vi "svpo_Average Array (complex).vi"(6 "averages completed in":dbl, 7 "restart averaging":bool, 8 "exponential weight (10 %)":dbl=10.0 min=0.0 max=100.0 step=5.0, 9 "weighting mode":enum16{"Linear", "Exponential"}(ring), 10 "array":cdb[](array[numeric]) format="%.2p", 11 "previous average array":cdb[](array[numeric]) format="%.2p") -> (2 "averages completed out":dbl, 3 "average array":cdb[](array[numeric]) format="%.2p")   [LabVIEW 2017]
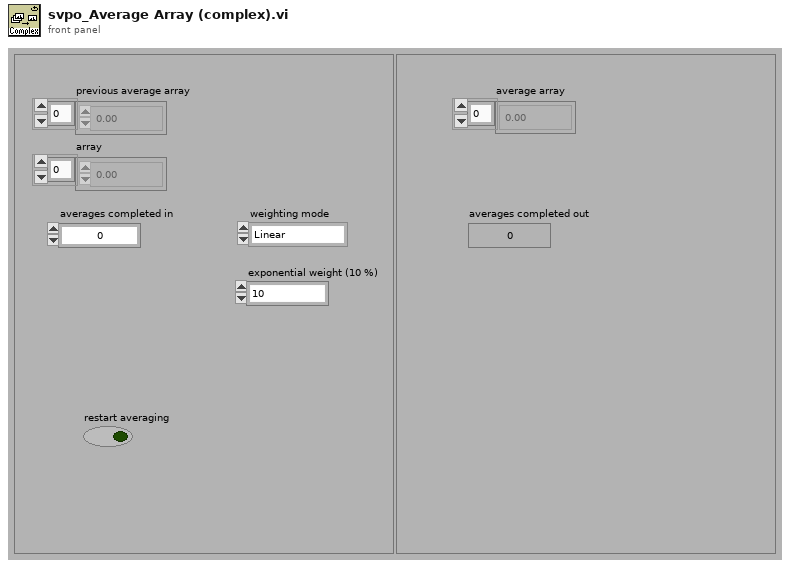
[diagram p1: front panel]
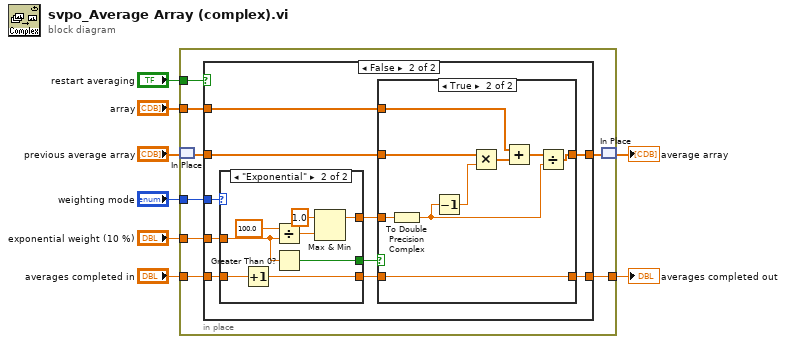
[diagram p0: block diagram]
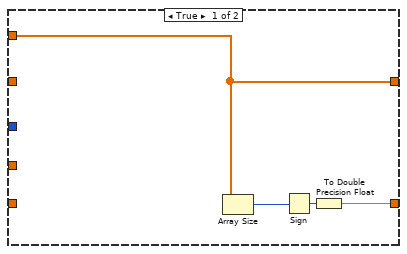
[diagram p2: hidden frame]
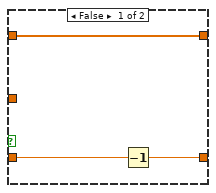
[diagram p3: hidden frame]
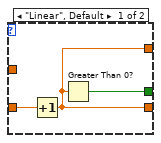
[diagram p4: hidden frame]
diagram:
  n1 = in-place {
    in-place-border: "array" -> [w16]
    in-place-border: "exponential weight (10 %)" -> [w15]
    in-place-border: "weighting mode" -> [w14]
    in-place-border: "averages completed in" -> [w13]
    in-place-border: [w12] -> w4
    in-place-border: "restart averaging" -> [w11]
    n2 = in-place-match #1("previous average array") -> (w10:cdb[])
    n3 = case shown="False" w11 {
      tunnel: w16 -> [w20 w29]
      tunnel: [w20 w24] -> w9
      tunnel: [w19 w22] -> w12
      tunnel: w10 -> [_ w28]
      tunnel: w15 -> [_ w27]
      tunnel: w14 -> [_ w26]
      tunnel: w13 -> [_ w25]
      frame True {
        n4 = Array Size(array=w20) -> (size(s)=w18:i32)
        n5 = Sign(1:w18) -> (0:w17:i32)
        n6 = To Double Precision Float(number=w17) -> (double precision float=w19:dbl)
      }
      frame False {
        n7 = case shown="\"Exponential\"" w26 {
          tunnel: w25 -> [w45 w52]
          tunnel: [w43 w53] -> w21
          tunnel: [w43 w46] -> w30
          tunnel: w27 -> [_ w48]
          tunnel: [w44 w47] -> w23
          frame "Linear", Default {
            n8 = Increment(x=w45) -> (x+1=w43:dbl)
            n9 = Greater Than 0?(x=w43) -> (x > 0?=w44:bool)
          }
          frame "Exponential" {
            n10 = Increment(x=w52) -> (x+1=w53:dbl)
            n11 = Divide(x=100.0, y=w48) -> (x/y=w51:dbl)
            n12 = Greater Than 0?(x=w48) -> (x > 0?=w47:bool)
            n13 = Max & Min(x=1.0 ("lower limit"), y=w51) -> (max(x,y)=w46:dbl)  [unwired: 1 out]
          }
        }
        n14 = case shown="True" w23 {
          tunnel: w30 -> [_ w35]
          tunnel: w29 -> [_ w40]
          tunnel: w28 -> [w33 w39]
          tunnel: [w33 w38] -> w24
          tunnel: [w31 w37] -> w22
          tunnel: w21 -> [w32 w37]
          frame False {
            n15 = Decrement(x=w32) -> (x-1=w31:dbl)
          }
          frame True {
            n16 = To Double Precision Complex(1:w35) -> (0:w34:cdb)
            n17 = Decrement(x=w34) -> (x-1=w36:cdb)
            n18 = Multiply(x=w39, y=w36) -> (x*y=w41:cdb[])
            n19 = Add(x=w40, y=w41) -> (x+y=w42:cdb[])
            n20 = Divide(x=w42, y=w34) -> (x/y=w38:cdb[])
          }
        }
      }
    }
    n21 = in-place-match #1(w9) -> (→"average array":cdb[])
  }
  "averages completed out" <- w4
